vi "_Add App.vi"(8 "error in (no error)":errorcluster, 11 "picoG in":refnum<class "picoG.lvclass">) -> (0 "error out":errorcluster, 3 "picoG out":refnum<class "picoG.lvclass">)   [LabVIEW 2020, in "PicoG-App.lvlib" / "picoG.lvclass"]
uses:
  picoG.lvclass
  picoG.lvclass/picoG.ctl
  ViaApp/ViaApp.lvclass
  App Watcher/App Watcher.lvclass
  AppListPanel/AppListPanel.lvclass
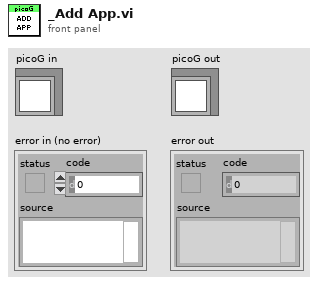
[diagram p1: front panel]
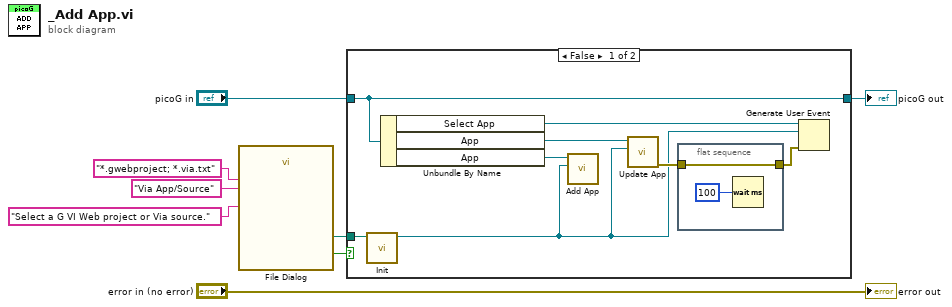
[diagram p0: block diagram]
diagram:
  n1 = call "File Dialog"("prompt"="Select a G VI Web project or Via source.", "pattern (all files)"="*.gwebproject; *.via.txt", "pattern label"="Via App/Source") -> ("selected path"=w2:path, "cancelled"=w3:bool)  [unwired: 9 in, 2 out]
  n2 = case shown="False" w3 {
    tunnel: "picoG in" -> [w12 w19]
    tunnel: w2 -> [w16 _]
    tunnel: [w12 w19] -> w1
    frame False {
      n3 = call "Init.vi"("Path"=w16) -> ("ViaApp out"=w10:refnum<class "ViaApp.lvclass">)  [unwired: 9 in, 1 out]
      n4 = Unbundle By Name(w12) -> ("Select App"=w13:refnum<user-event>, "App"=w14:refnum<class "AppListPanel.lvclass">, "App"=w15:refnum<class "App Watcher.lvclass">)
      n5 = call "Add App.vi"("ViaApp"=w10, "App Watcher in"=w15) -> ()  [unwired: 8 in, 2 out]
      n6 = call "Update App.vi"("ViaApp"=w10, "AppListPanel in"=w14) -> ("error out"=w11:errorcluster)  [unwired: 8 in, 1 out]
      n7 = flat-sequence {
        tunnel: w11 -> [w18]
        tunnel: [w18] -> w9
        frame #0 {
          n8 = Wait (ms)(milliseconds to wait=u32 100) -> ()  [unwired: 1 out]
        }
      }
      n9 = Generate User Event(user event=w13, event data cluster=w10, error in=w9) -> ()  [unwired: 1 in, 2 out]
    }
    frame True {
    }
  }
  "picoG out" <- w1
  "error out" <- "error in (no error)"
